vi "Scalogram with Analytic Wavelet Transform.vi"() -> ()   [LabVIEW 2023]
doc: "This example shows how to perform time-frequency analysis on a nonstationary signal by computing the analytic wavelet transform. The frequency of the HypChirp signal is modulated by a hyperbolic function. By computing the analytic wavelet transform, you can obtain fine frequency resolution and fine time resolution at low frequencies and high frequencies, respectively. This example uses the WA Analytic Wavelet Transform VI.\n\n<b>Instructions:</b>\n1) Run this VI.\n2) Observe the <b>Scalogram</b> of the signal by using different settings."
uses:
  <vilib>/addons/Wavelet Analysis/continuous wavelet transform.llb/WA Analytic Wavelet Transform (Waveform).vi
  <vilib>/addons/Wavelet Analysis/misc.llb/WA Configure Scalogram Indicator (Predefined Color Table, Complex).vi
  <vilib>/addons/_Advanced Signal Processing/NI_AdvSigProcWA.lvlib
panel:
  in  "Data":u16(ring)=114 items=["1D Example Data"=100, "-"=101, "Doppler"=102, "HOP"=103, "TF Sine"=104, "Noisy Doppler"=105, "Sea Temperature"=106, "Sp500"=107, "Power Line"=108, "Engine Knocking"=109, "HeaviSine"=110, "Bumps"=111, "Blocks"=112, "Piece Regular"=113, "HypChirps"=114, "LinChirps"=115, "Chirps"=116, "Piece Polynomial"=117, "ECG"=131, "-"=118, "2D Example Data"=119, "-"=120, "Finger Print (Image)"=121, "Iris Flower (Image)"=122, "Mammogram (Image)"=123, "Lake (Image)"=127, "Two Can 1 (Image)"=132, "Two Can 2 (Image)"=133, "Camera Man (Image)"=134]
  in  "Normalization":u16(ring) items=["Energy", "Amplitude"]
  in  "Time steps":i32=-1
  in  "stop":bool
  out "Scalogram":dbl[][](graph)
  out "Signal":waveform(dbl)(graph)
  in  "Scale Sampling Method":u16(ring) items=["Even freq", "Even scale"]
  in  "Scales":i32=128 min=1
  # "Overview: Shows how to perform time-frequency analysis on a nonstationary signal by computing the analytic wavelet transform. \nRequirements: LabVIEW Full Development System, Advanced Signal Processing Toolkit\nInstructions: \n1. Run this VI.\n2. Observe the Scalogram of the signal by using different settings.\n3. Click Stop to stop the VI."
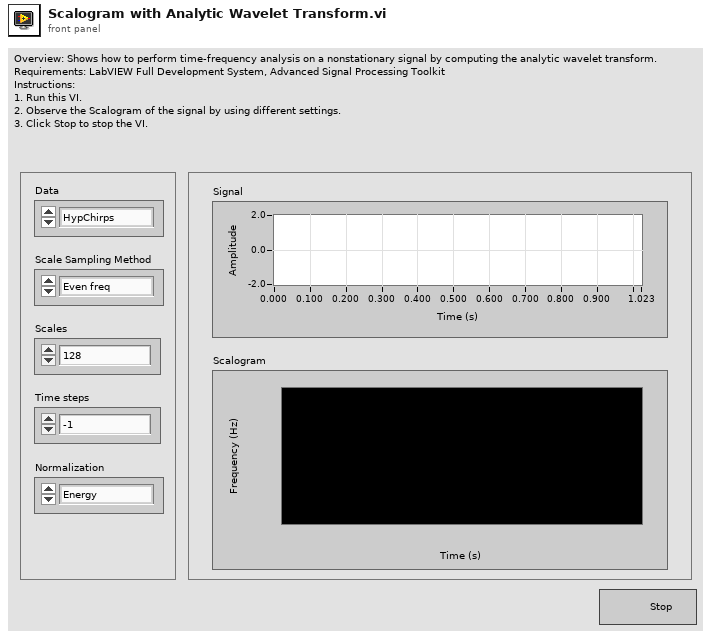
[diagram p1: front panel]
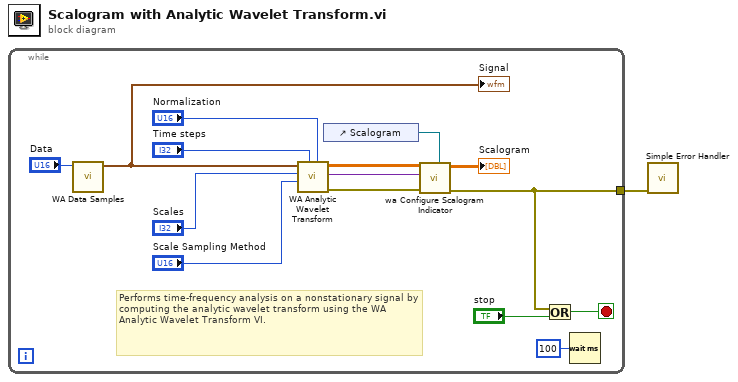
[diagram p0: block diagram]
diagram:
  n1 = while {
    tunnel: [w3] -> w1
    stop <- w8 stop-if-true
    # "Performs time-frequency analysis on a nonstationary signal by computing the analytic wavelet transform using the WA Analytic Wavelet Transform VI."
    n2 = call <vilib>:"WA Data Samples.vi"("data"="Data") -> ("signal"=w15:waveform(dbl))  [unwired: 10 out]
    "Signal" <- w15
    n3 = call-poly <vilib>:"WA Analytic Wavelet Transform.vi"("normalization"="Normalization", "time steps"="Time steps", "scale sampling method"="Scale Sampling Method", "scales"="Scales", "signal"=w15) -> ("error out"=w13:errorcluster, "scale info"=w14:variant, "AWT coef"=w6:cdb[][])  [unwired: 1 in, 3 out]
    n4 = control-ref of="Scalogram"() -> (w11:refnum<vi>)
    n5 = call-poly <vilib>:"wa Configure Scalogram Indicator.vi"("reference of scalogram indicator"=w11, "error in (no error)"=w13, "scale info"=w14, "AWT coef"=w6) -> ("error out"=w3:errorcluster, "scalogram indicator"=→"Scalogram":dbl[][])  [unwired: 4 in, 2 out]
    n6 = Or(x=w3, y="stop") -> (x .or. y?=w8:bool)
    n7 = Wait (ms)(milliseconds to wait=u32 100) -> ()  [unwired: 1 out]
  }
  n8 = call <vilib>:"Simple Error Handler.vi"("error in (no error)"=w1) -> ()  [unwired: 1 in, 8 out]
